vi "Drive Play Path.vi"(7 "Description":string, 8 "Command Info In":T2, 11 "Auto":T1) -> (0 "Command Info Out":T2)   [LabVIEW 2020]
doc: "Often used for joystick control, this VI checks to see that the joystick axes are outside the deadband and updates the motors appropriately."
uses:
  <vilib>/Rock Robotics/WPI/Framework/Command Status Info.ctl
  <vilib>/Rock Robotics/WPI/Framework/Completion Status.ctl
  <vilib>/Rock Robotics/WPI/Framework/Completion Notifier.ctl
  Support Code/Auto/Auto.ctl
  Implementation/Drive Setpoints.ctl
  Implementation/Drive Operations.ctl
  Support Code/Teleop/Types/Swerve Mode.ctl
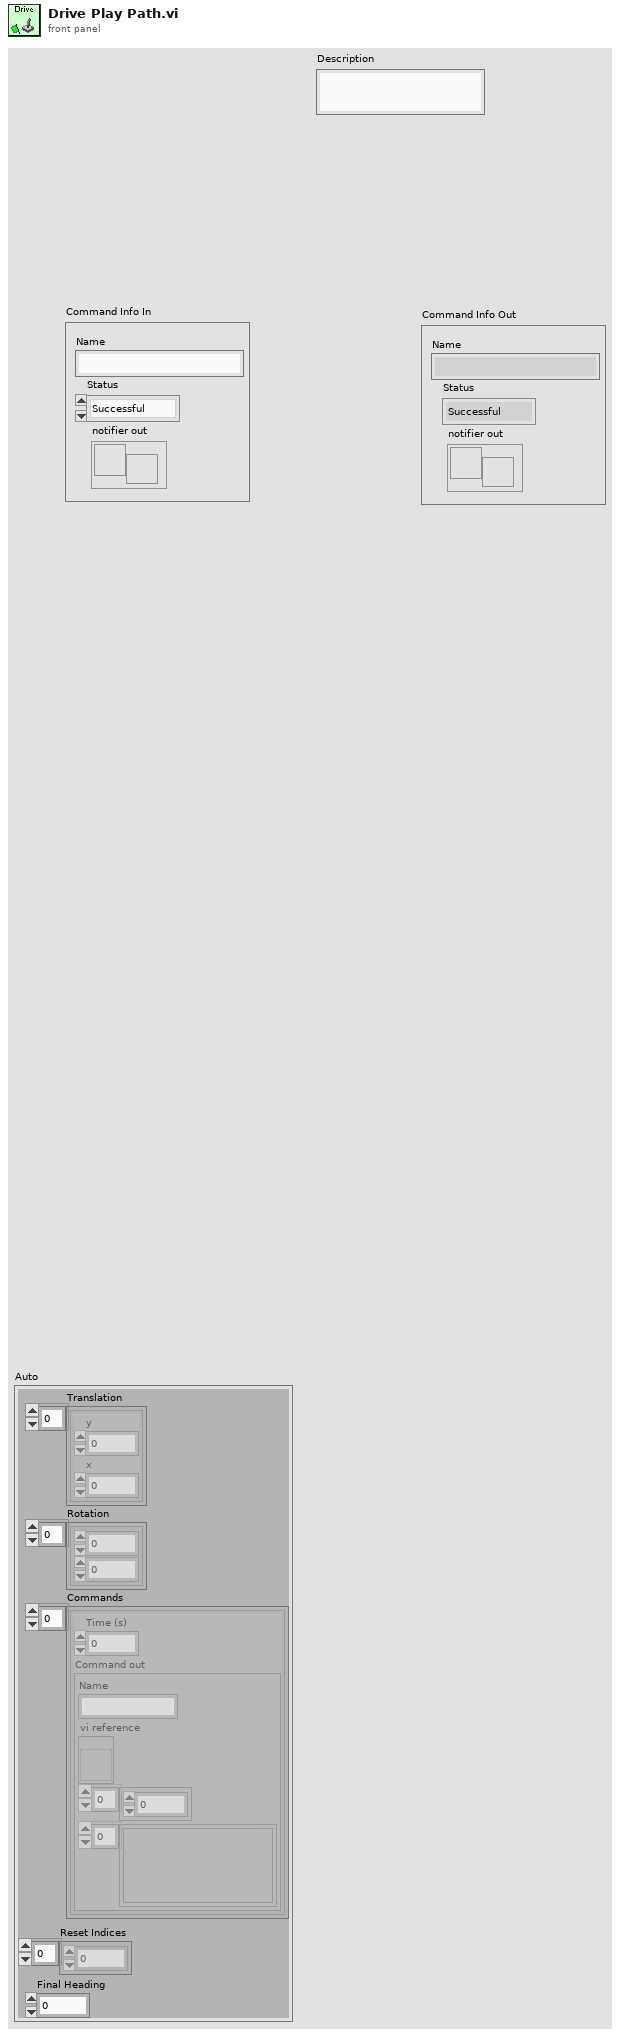
[diagram p1: front panel]
types:
  T1 = typedef "Auto.ctl" = cluster{"Translation":cluster{"y":dbl, "x":dbl}[], "Rotation":cluster{dbl, dbl}[], "Commands":cluster{"Time (s)":dbl, "Command out":cluster{"Name":string, "vi reference":refnum<vi>, i32[], variant[]}}[], "Reset Indices":i32[], "Final Heading":dbl}
  T2 = typedef "Command Status Info.ctl" = cluster{"Name":string, "Status":T3, "notifier out":T4}
  T3 = typedef "Completion Status.ctl" = enum16{"Successful", "Aborted", "Incomplete"}
  T4 = typedef "Completion Notifier.ctl" = refnum<notifier>
  T5 = typedef "Drive Operations.ctl" = enum16{"Reserve", "Read Current", "Immediate", "Calibrate", "Play Path", "Immediate MM", "Set Schtuff"}
  T6 = typedef "Drive Setpoints.ctl" = cluster{"Operation":T5, "Trans Vel":cluster{"x":dbl, "y":dbl}, "Rot Vel":cluster{"omega":dbl}, "reset pods":bool, "Limits":cluster{"Trans Vel":dbl, "Rot Vel":dbl, "Trans Acc":dbl, "Rot Acc":dbl, "Trans De-Acc":dbl, "Rot De-Acc":dbl}, "Drive Mode":T7, "Auto":T1}
  T7 = typedef "Swerve Mode.ctl" = enum16{"Robot Centric", "Field Centric", "Robot Centric (Backwards)"}
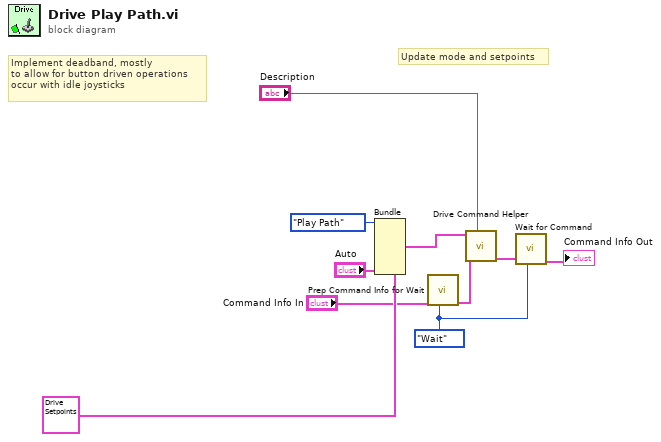
[diagram p0: block diagram]
diagram:
  w3 = enum16{"Start", "Wait"}."Wait" ("Synchronication")
  # "Implement deadband, mostly\nto allow for button driven operations\noccur with idle joysticks"
  # "Update mode and setpoints"
  n1 = Bundle(cluster=T6 {"Operation"=enum."Play Path", "Trans Vel"={"x"=0.0, "y"=0.0}, "Rot Vel"={"omega"=0.0}, "reset pods"=FALSE, "Limits"={"Trans Vel"=0.0, "Rot Vel"=0.0, "Trans Acc"=0.0, "Rot Acc"=0.0, "Trans De-Acc"=0.0, "Rot De-Acc"=0.0}, "Drive Mode"=enum."Robot Centric", "Auto"={"Translation"=[], "Rotation"=[], "Commands"=[], "Reset Indices"=[], "Final Heading"=0.0}} ("SubSystem Data"), "Operation"=Drive_Operations."Play Path", "Auto"="Auto") -> (w8:T6)  [unwired: 5 in]
  n2 = call <vilib>:"Prep Command Info for Wait.vi"("Synchronication"=w3, "Command Info"="Command Info In") -> ("Command Info"=w6:T2)  [unwired: 8 in, 1 out]
  n3 = call "Drive Command Helper.vi"("Description"="Description", "Command Info In"=w6, "SubSystem Data"=w8) -> ("Command Info Out"=w5:T2)  [unwired: 6 in, 2 out]
  n4 = call <vilib>:"Wait for Command.vi"("Synchronication"=w3, "Command Info in"=w5) -> ("Command Info out"=→"Command Info Out":T2)  [unwired: 9 in]
